vi "Station.GetStatus.vi"(8 "error in (no error)":errorcluster, 11 "Station.ID":string) -> (0 "error out":errorcluster, 2 "timed out?":bool, 3 "Station.Status":T1)   [LabVIEW 2015, in "Shared.lvlib"]
uses:
  Shared.lvlib
  Execution GUI/Types/Stimulus.Status.ctl
  Execution GUI/Types/Execution.SequenceState.ctl
  <vilib>/NI/AMC/Create Single Message.vi
  <vilib>/NI/AMC/Update Message Routing Info.vi
  <vilib>/NI/AMC/Read Termination Message.vi
  <vilib>/NI/AMC/Send Message.vi
  <vilib>/NI/AMC/Globals.vi
  <vilib>/NI/AMC/AMC.lvlib
  Execution GUI/Single Station Execution.lvlib
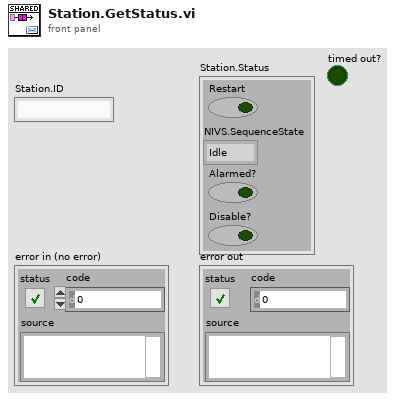
[diagram p1: front panel]
types:
  T1 = typedef "Single Station Execution.lvlib/Stimulus.Status.ctl" = cluster{"Restart":bool, "NIVS.SequenceState":T2, "Alarmed?":bool, "Disable?":bool}
  T2 = typedef "Single Station Execution.lvlib/Execution.SequenceState.ctl" = enum16{"Idle", "Initializing", "Running", "Paused", "Finalizing", "Complete"}
  T3 = typedef "AMC.lvlib/Message Queue.ctl" = refnum<queue>
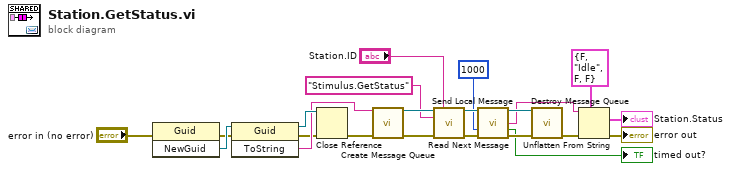
[diagram p0: block diagram]
diagram:
  n1 = invoke class="Guid" method="NewGuid"(error in="error in (no error)") -> (error out=w4:errorcluster, "NewGuid"=w7:refnum<k24>)  [unwired: 2 in, 1 out]
  n2 = invoke class="Guid" method="ToString"(reference=w7, error in=w4) -> (reference out=w6:refnum<k24>, error out=w3:errorcluster, "ToString"=w5:string)  [unwired: 1 in]
  n3 = Close Reference(reference=w6, error in (no error)=w3) -> (error out=w1:errorcluster)
  n4 = call <vilib>:"Create Message Queue.vi"("message queue name"=w5, "error in"=w1) -> ("message queue out"=w18:T3, "error out"=w11:errorcluster)  [unwired: 12 in]
  n5 = call <vilib>:"Send Local Message.vi"("message queue in"=w18, "receiver process (\"\" - local)"="Station.ID", "message name"="Stimulus.GetStatus" ("message value"), "error in"=w11) -> ("message queue out"=w17:T3, "error out"=w16:errorcluster)  [unwired: 9 in, 1 out]
  n6 = call <vilib>:"Read Next Message.vi"("message queue in"=w17, "timeout (1 ms)"=1000, "error in"=w16) -> ("message queue out"=w14:T3, "message value"=w10:string, "timed out?"=→"timed out?":bool, "error out"=w13:errorcluster)  [unwired: 5 in, 4 out]
  n7 = call <vilib>:"Destroy Message Queue.vi"("message queue in"=w14, "error in"=w13) -> ("error out"=w20:errorcluster)  [unwired: 11 in, 2 out]
  n8 = Unflatten From String(type=T1 {"Restart"=FALSE, "NIVS.SequenceState"=enum."Idle", "Alarmed?"=FALSE, "Disable?"=FALSE} ("cluster"), binary string=w10, error in (no error)=w20) -> (value=→"Station.Status":T1, error out=→"error out":errorcluster)  [unwired: 2 in, 1 out]
